vi "AlazarBusy.vi"(0 "Handle":u64, 1 "error in (no error)":errorcluster) -> (2 "Handle":u64, 3 "Busy":bool, 4 "Return Code":u32, 5 "error out":errorcluster)   [LabVIEW 2009]
doc: "Determine if an acquisition to on-board memory is in progress."
uses:
  ATSApi.dll
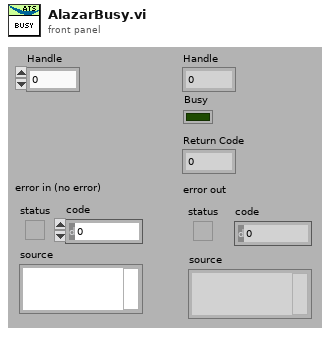
[diagram p1: front panel]
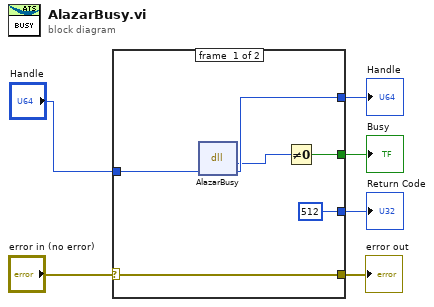
[diagram p0: block diagram]
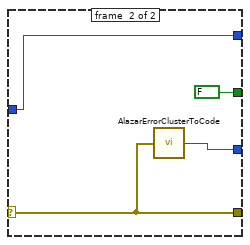
[diagram p2: hidden frame]
diagram:
  n1 = case shown="No Error" "error in (no error)" {
    selector: "error in (no error)" -> [w9 w16]
    tunnel: [w9 w16] -> w5
    tunnel: [u32 512 w15] -> w4
    tunnel: "Handle" -> [w12 w14]
    tunnel: [w11 w14] -> w2
    tunnel: [w7 FALSE] -> w1
    frame #0 {
      n2 = dll-call lib="ATSApi.dll" fn="AlazarBusy"("handle"=w12) -> ("return type"=w8:u32, "handle"=w11:u64)  [unwired: 3 in, 2 out]
      n3 = Not Equal To 0?(x=w8) -> (x != 0?=w7:bool)
    }
    frame #1 {
      n4 = call "AlazarErrorClusterToCode.vi"("error in (no error)"=w16) -> ("Error Code"=w15:u32)
    }
  }
  "Handle" <- w2
  "error out" <- w5
  "Return Code" <- w4
  "Busy" <- w1
